vi "Run Tests.vi"() -> ()   [LabVIEW 2023]
uses:
  <vilib>/addons/_JKI Toolkits/Caraya/classes/Assert/Assert Not Error.vi
  <vilib>/addons/_JKI Toolkits/Caraya/classes/Test/Test.lvclass
  <vilib>/addons/_JKI Toolkits/Caraya/classes/Assert/Assert.lvclass
panel:
  out "error out":errorcluster
  in  "error in (no error)":errorcluster
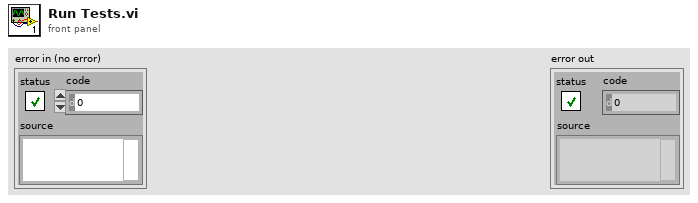
[diagram p1: front panel]
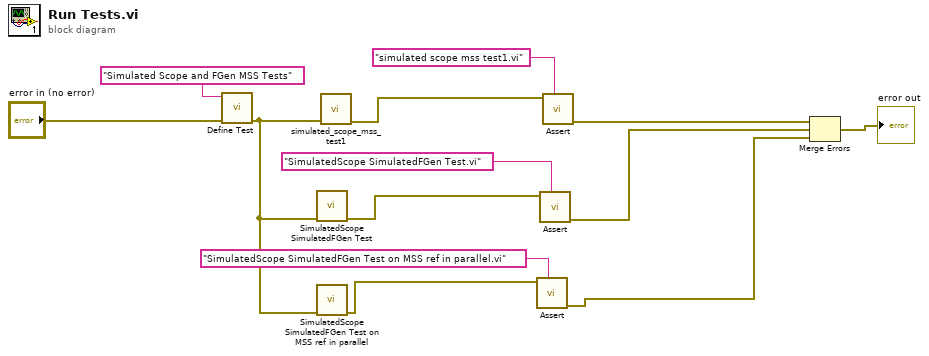
[diagram p0: block diagram]
diagram:
  n1 = call <vilib>:"Define Test.vi"("error in (no error)"="error in (no error)", "Label (VI Title)"="Simulated Scope and FGen MSS Tests") -> ("error out"=w4:errorcluster)  [unwired: 8 in, 1 out]
  n2 = call "SimulatedScope SimulatedFGen Test.vi"("Error In"=w4) -> ("Error Out"=w10:errorcluster)  [unwired: 10 in]
  n3 = call "SimulatedScope SimulatedFGen Test on MSS ref in parallel.vi"("Error In"=w4) -> ("Error Out"=w1:errorcluster)  [unwired: 10 in]
  n4 = call "simulated_scope_mss_test1.vi"("Error In"=w4) -> ("Error Out"=w12:errorcluster)  [unwired: 10 in]
  n5 = call-poly <vilib>:"Assert.vi"("Label"="SimulatedScope SimulatedFGen Test on MSS ref in parallel.vi", "Not Error?"=w1) -> ("error out"=w2:errorcluster)  [unwired: 8 in, 1 out]
  n6 = call-poly <vilib>:"Assert.vi"("Label"="SimulatedScope SimulatedFGen Test.vi", "Not Error?"=w10) -> ("error out"=w8:errorcluster)  [unwired: 8 in, 1 out]
  n7 = call-poly <vilib>:"Assert.vi"("Label"="simulated scope mss test1.vi", "Not Error?"=w12) -> ("error out"=w13:errorcluster)  [unwired: 8 in, 1 out]
  n8 = Merge Errors(w13, w8, w2) -> (→"error out":errorcluster)
